vi "ep_Initialize Calibration Instrument.vi"(11 "error in (no error)":errorcluster) -> (15 "error out":errorcluster)   [LabVIEW 2012]
panel:
  in  "VISA resource name":refnum<visa-resource-name>
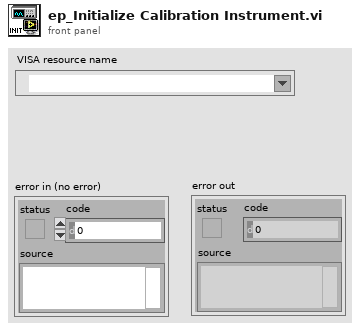
[diagram p1: front panel]
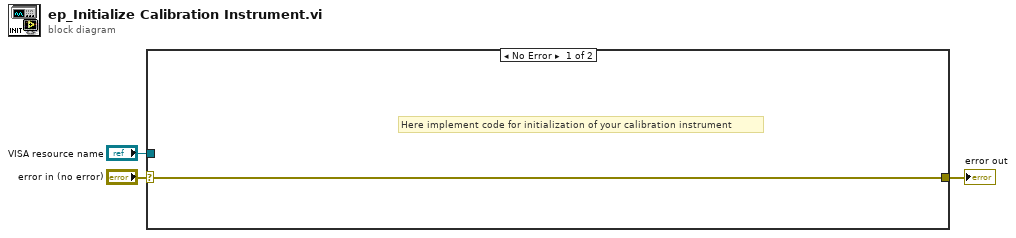
[diagram p0: block diagram]
diagram:
  n1 = case shown="No Error" "error in (no error)" {
    selector: "error in (no error)" -> [w4 w5]
    tunnel: "VISA resource name" -> [_ _]
    tunnel: [w4 w5] -> w2
    frame No Error {
      # "Here implement code for initialization of your calibration instrument"
    }
    frame Error {
    }
  }
  "error out" <- w2
